vi "Detector_senales_simp.vi"() -> ()   [LabVIEW 2017]
panel:
  out "Conteo":bool
  in  "Boolean 2":bool
  out "Waveform Chart":dbl(graph)
  in  "stop 2":bool
  out "Numeric Indicator 2":dbl
  out "Numeric Indicator":dbl
  in  "Boolean":bool
  in  "stop":bool
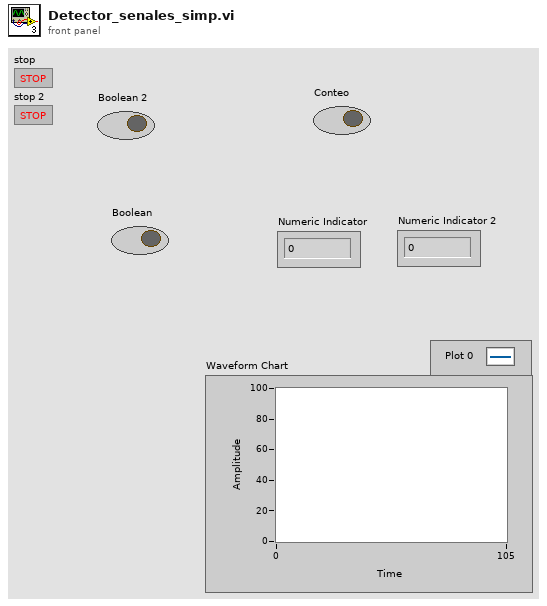
[diagram p1: front panel]
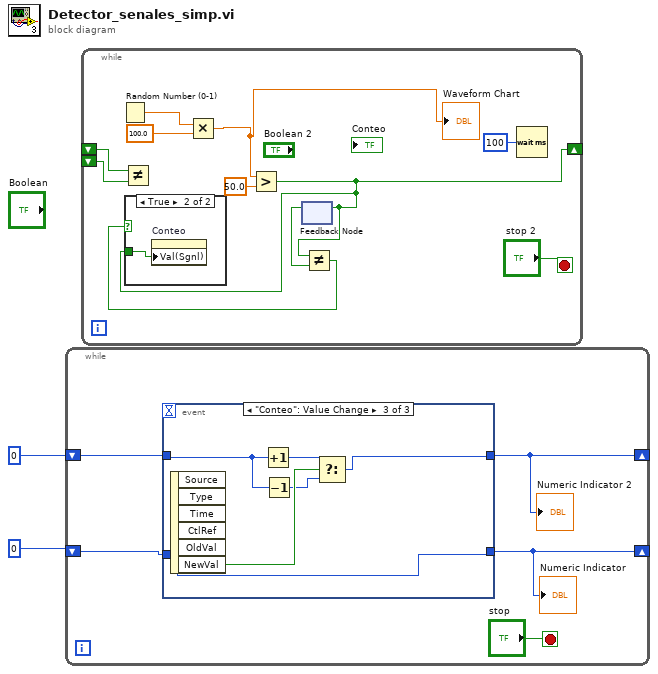
[diagram p0: block diagram]
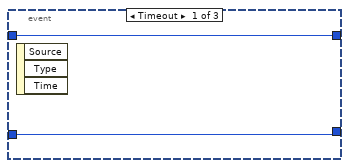
[diagram p3: hidden frame]
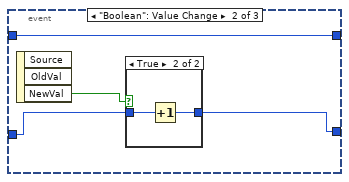
[diagram p4: hidden frame]
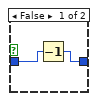
[diagram p5: hidden frame]
diagram:
  n1 = while {
    shift-right: [w4] -> _
    shift-left: 0 -> [w6]
    shift-right: [w3] -> _
    shift-left: 0 -> [w7]
    stop <- "stop" stop-if-true
    n2 = event shown="[2] \"Conteo\": Value Change" {
      selector: _ -> [_ _ _]
      dyn-events: _ -> [_ _ _]
      timeout: _ -> [_ _ _]
      tunnel: w7 -> [w9 w13 w19]
      tunnel: w6 -> [w8 w11 w23]
      tunnel: [w8 w10 w23] -> w4
      tunnel: [w9 w13 w18] -> w3
      event Timeout {
        n3 = event-data() -> ()  [unwired: 1 in, 3 out]
      }
      event "Boolean": Value Change {
        n4 = event-data() -> ("NewVal"=w12:bool)  [unwired: 1 in, 2 out]
        n5 = case shown="True" w12 {
          tunnel: w11 -> [w15 w17]
          tunnel: [w14 w16] -> w10
          frame False {
            n6 = Decrement(x=w15) -> (x-1=w14:i32)
          }
          frame True {
            n7 = Increment(x=w17) -> (x+1=w16:i32)
          }
        }
      }
      event "Conteo": Value Change {
        n8 = event-data() -> ("NewVal"=w22:bool)  [unwired: 1 in, 5 out]
        n9 = Increment(x=w19) -> (x+1=w21:i32)
        n10 = Decrement(x=w19) -> (x-1=w20:i32)
        n11 = Select(t=w21, s=w22, f=w20) -> (s? t:f=w18:i32)
      }
    }
    "Numeric Indicator" <- w4
    "Numeric Indicator 2" <- w3
  }
  n12 = while {
    shift-right: [w26] -> _
    shift-left: _ -> [w27]
    shift-left: _ -> [w28]
    stop <- "stop 2" stop-if-true
    n13 = Random Number (0-1)() -> (number: 0 to 1=w34:dbl)
    n14 = Not Equal?(x=w27, y=w28) -> ()  [unwired: 1 out]
    n15 = Multiply(x=w34, y=100.0) -> (x*y=w30:dbl)
    "Waveform Chart" <- w30
    n16 = Greater?(x=w30, y=50.0) -> (0:w26:bool)
    n17 = feedback-in #1(w26) -> ()
    n18 = feedback #1() -> (w24:bool)  [unwired: 1 in]
    n19 = Not Equal?(x=w26, y=w24) -> (x != y?=w25:bool)
    n20 = case shown="True" w25 {
      tunnel: w26 -> [_ w35]
      frame False {
      }
      frame True {
        n21 = property on="Conteo" class="Bool (strict)"("Val(Sgnl)"=w35) -> ()  [unwired: 2 in, 2 out]
      }
    }
    n22 = Wait (ms)(milliseconds to wait=u32 100) -> ()  [unwired: 1 out]
  }
